vi "Tetra_Globals.vi"() -> ()   [LabVIEW 2018]
panel:
  in  "Tab Control":T1(tab)
  out "atten(code)ary (ro)":i32[](array[numeric])=[31, 5, 63, 63]
  out "Atten0":dbl
  out "Atten1-3":dbl
  out "txatten-sel":i32=1
  out "cmd;":string
  out "TX_PORT":i32=1
  out "TX_FILTER":i32=2
  in  "PASS_SYS-STD(T)":bool caption="Place entry into test log"
  in  "Prod_Mode(T)":bool=TRUE caption="Place entry into test log"
  out "-ssid":string
  out "BarCodeESN":string
  out "RevC(t)":bool
  out "Revision":string
  out "comport":refnum<visa-resource-name>="COM4"
  out "ESN":string
  out "RX_N_FREQ_LIST":dbl[](array[numeric])
  out "Gantry_Z":dbl
  out "TestBench_ID":string
  out "TEMP(t)":bool
  out "RX_INPUT_OFFSET":dbl[][](array[numeric])
  out "FSPL_CAL":dbl[][](array[numeric])
  out "HORN_CAL":dbl[][](array[numeric])
  out "RF_CAL":dbl[][](array[numeric])
  out "OUT_CAL":dbl[][](array[numeric])
  out "REF_CAL":dbl[][](array[numeric])
  out "WAM_Prod_limits":cluster{"names":string, "limits":dbl}[](array[cluster])
  out "NF_MASK":dbl[][](array[numeric])
  out "Ver_Tags(ary)":string[](array[string])
  out "TraceFilePath":path
  out "s11_path":path
  out "-dynamic (t)":bool
  out "RunAM_Init(T)":bool
  out "RundynamicMode_Init(T)":bool
  in  "Use Serial log(T)":bool caption="Boolean 9"
  in  "Ser log Folder":path=path "C:/RageATE/Automated Tests/Tetra WAM/PRODUCTION/setup files/Tetra_PROD_Instruments.csv" caption="Test Parameters File"
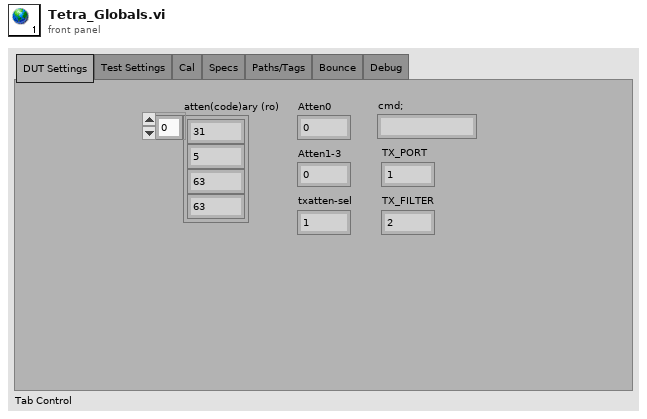
[diagram p1: front panel]
types:
  T1 = enum32{"DUT Settings", "Test Settings", "Cal", "Specs", "Paths/Tags", "Bounce", "Debug"}
diagram:
